vi "cm2nm_add_new_sample_point_to_session_array.vi"(4 "Sample Set":T2, 6 "Enter New Point":T1) -> (0 "XY_graphOut":cluster{dbl[], dbl[]}[](array[cluster]), 1 "NewPoint":T1={"MetaDataFile"=path "", "X"=nan, "Y"=nan, "Z"=0.0, "Group"=0, "Rotation"=0.0, "Fiducial"=FALSE, "Magnification"=0.0, "Working_Distance"=0.0, "Notes"="", "Location Name/ID"="", "OtherRelatedDataFiles"=[], "Available"=FALSE}, 2 "SetIndexOfarrytoEnd":i32[](array[numeric]), 3 "Sample Set Out":T2, 5 "Fiducial Count":u32[](array[colorbox]), 7 "List of Points":string[](array[string]))   [LabVIEW 2011]
uses:
  cm2nm_coordinate_information_v2.ctl
  cm2nm_sample_set.ctl
  Instrument_type_enum_v2.ctl
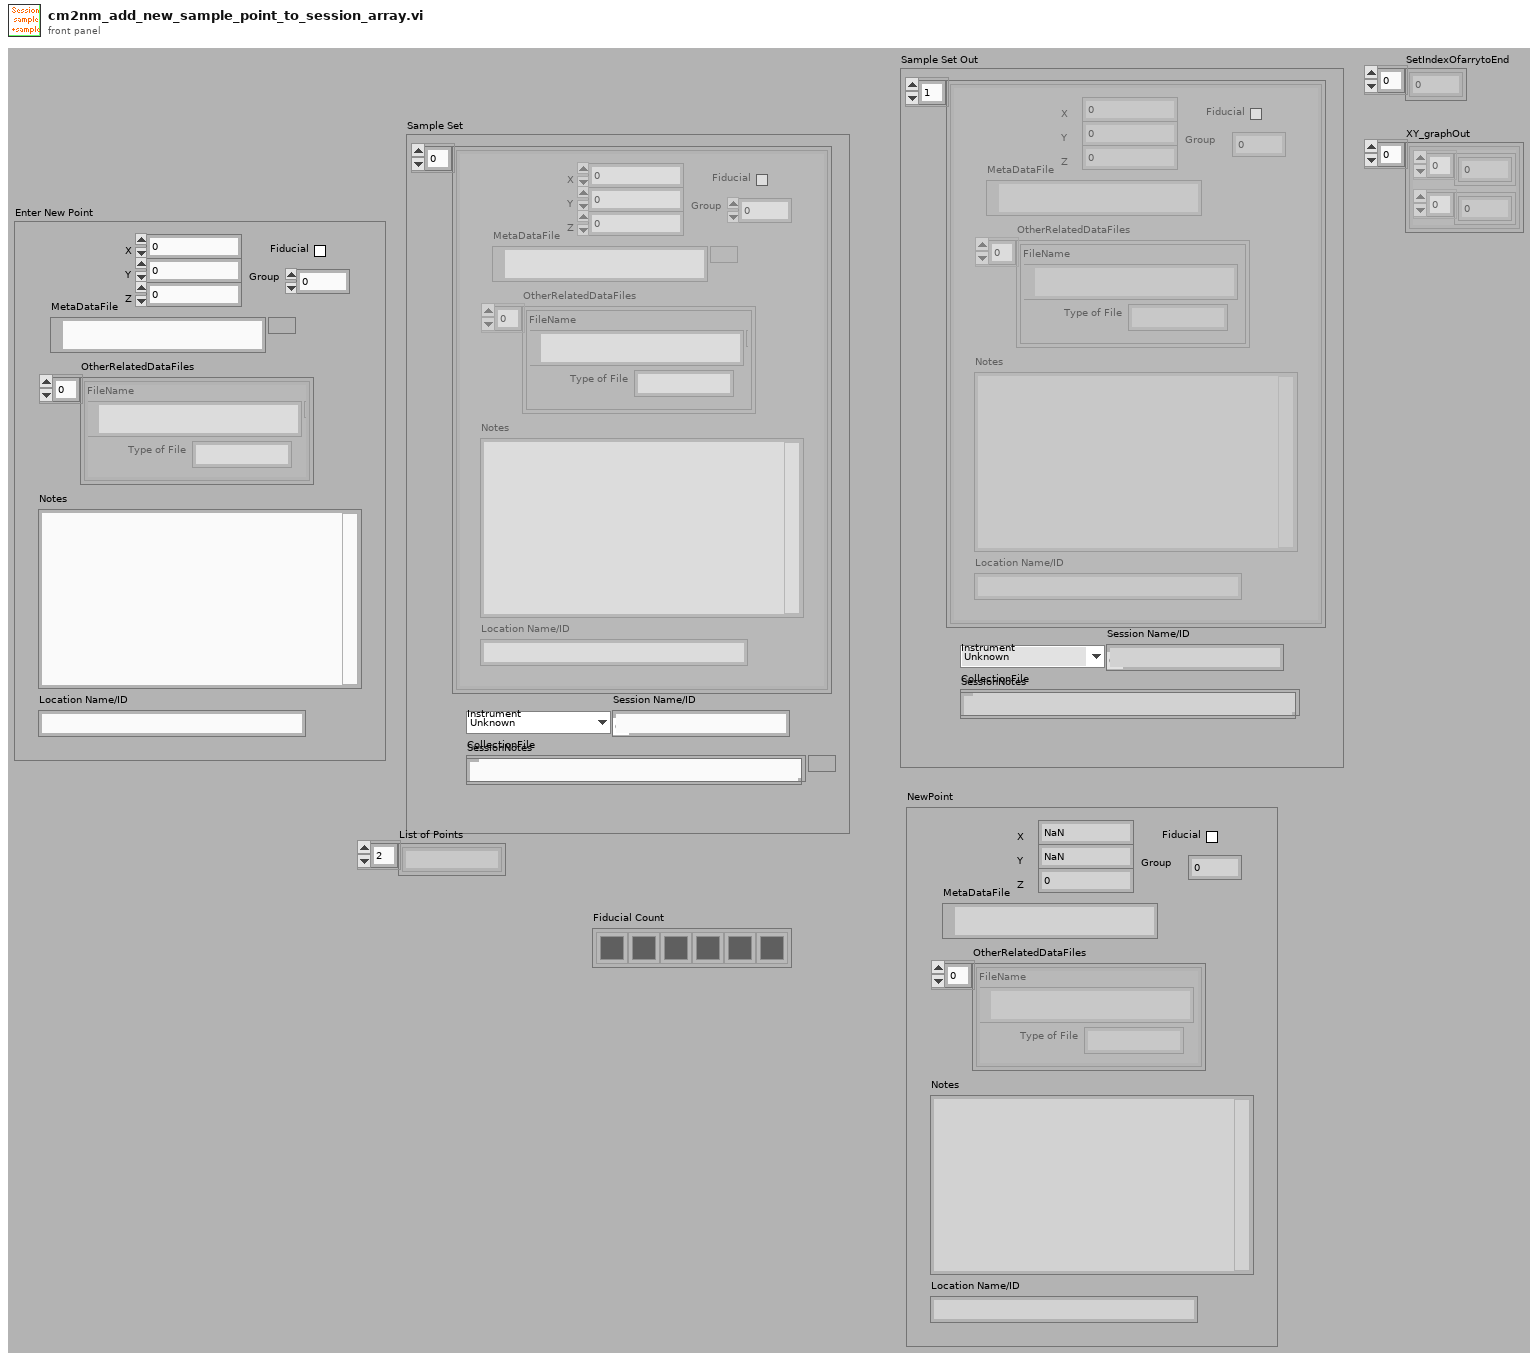
[diagram p1: front panel]
types:
  T1 = typedef "cm2nm_coordinate_information_v2.ctl" = cluster{"MetaDataFile":path, "X":dbl, "Y":dbl, "Z":dbl, "Group":i32, "Rotation":dbl[unit], "Fiducial":bool, "Magnification":dbl, "Working_Distance":dbl, "Notes":string, "Location Name/ID":string, "OtherRelatedDataFiles":cluster{"Type of File":string, "FileName":path}[], "Available":bool}
  T2 = typedef "cm2nm_sample_set.ctl" = cluster{"CollectionOfPoints":T1[], "Instrument":T3, "CollectionFile":path, "Session Name/ID":string, "SessionNotes":string}
  T3 = typedef "Instrument_type_enum_v2.ctl" = enum16{"Unknown", "Philips FEI SEM IRC", "JEOL 7000F EML_MFC", "MXRD MFC", "JEOL_EPMA"}
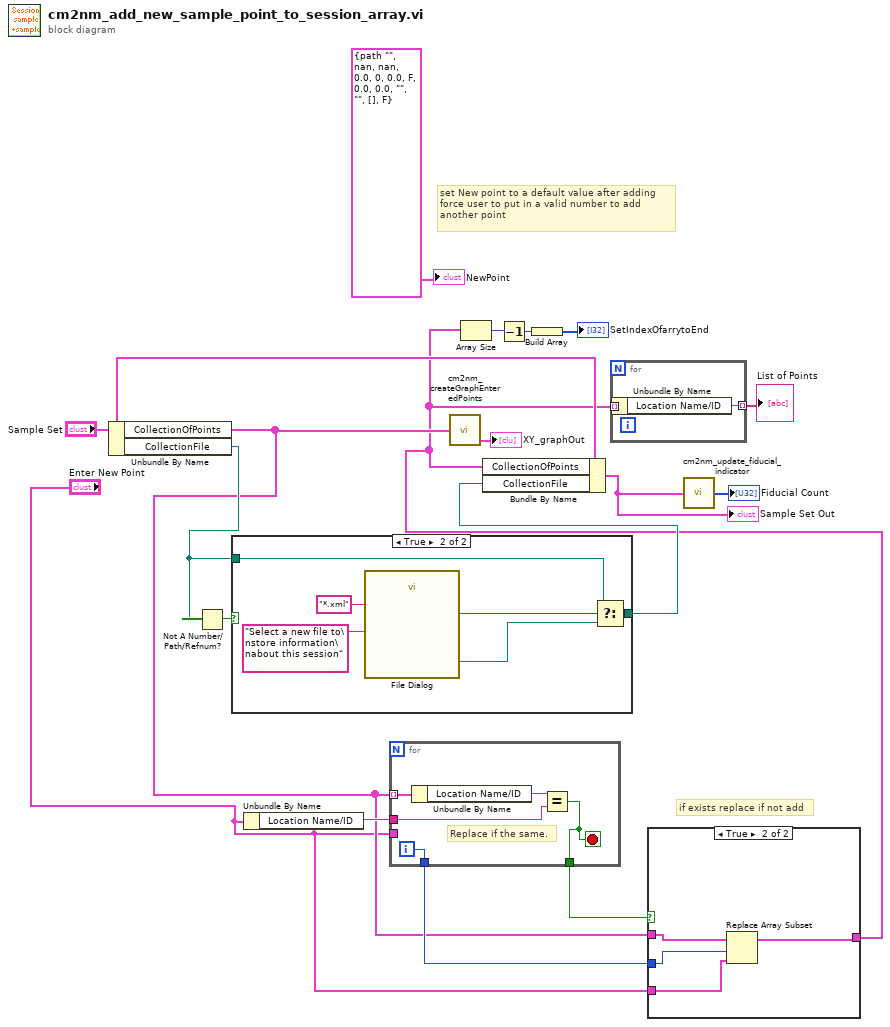
[diagram p0: block diagram]
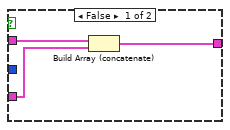
[diagram p2: hidden frame]
diagram:
  # "if exists replace if not add"
  # "set New point to a default value after adding\nforce user to put in a valid number to add\nanother point"
  n1 = Unbundle By Name("Sample Set") -> ("CollectionOfPoints"=w3:T1[], "CollectionFile"=w9:path)
  n2 = Not A Number/Path/Refnum?(number/path/refnum=w9) -> (NaN/Path/Refnum?=w10:bool)
  n3 = case shown="True" w10 {
    tunnel: w9 -> [w19 w20]
    tunnel: [w19 w21] -> w8
    frame False {
    }
    frame True {
      n4 = call "File Dialog"("prompt"="Select a new file to\nstore information\nabout this session", "pattern (all files)"="*.xml") -> ("selected path"=w22:path, "cancelled"=w23:bool)  [unwired: 5 in, 7 out]
      n5 = Select(t=w20, s=w23, f=w22) -> (s? t:f=w21:path)
    }
  }
  n6 = Unbundle By Name("Enter New Point") -> ("Location Name/ID"=w6:string)
  n7 = for {
    tunnel: w3 -> [w28] mode=indexing
    tunnel: w6 -> [w30]
    tunnel: "Enter New Point" -> [_]
    tunnel: [w27] -> w4
    tunnel: [w26] -> w5
    i -> [w27]
    stop <- w26 stop-if-true
    # "Replace if the same."
    n8 = Unbundle By Name(w28) -> ("Location Name/ID"=w29:string)
    n9 = Equal?(x=w29, y=w30) -> (x = y?=w26:bool)
  }
  n10 = call "cm2nm_createGraphEnteredPoints.vi"("EnteredPoints_in"=w3) -> ("XY_graphOut"=→"XY_graphOut":cluster{dbl[], dbl[]}[])
  n11 = case shown="True" w5 {
    tunnel: w4 -> [_ w36]
    tunnel: w3 -> [w33 w37]
    tunnel: "Enter New Point" -> [w32 w35]
    tunnel: [w31 w34] -> w1
    frame False {
      n12 = Build Array (concatenate)(w33, w32) -> (w31:T1[])
    }
    frame True {
      n13 = Replace Array Subset(array=w37, new element=w35, index=w36) -> (w34:T1[])
    }
  }
  n14 = Array Size(array=w1) -> (size(s)=w15:i32)
  n15 = Bundle By Name(cluster="Sample Set", "CollectionOfPoints"=w1, "CollectionFile"=w8) -> (w11:T2)
  "Sample Set Out" <- w11
  n16 = Decrement(x=w15) -> (x-1=w14:i32)
  n17 = Build Array(w14) -> (→"SetIndexOfarrytoEnd":i32[])
  n18 = for {
    tunnel: w1 -> [w39] mode=indexing
    tunnel: [w38] -> w7 mode=indexing
    n19 = Unbundle By Name(w39) -> ("Location Name/ID"=w38:string)
  }
  "List of Points" <- w7
  n20 = call "cm2nm_update_fiducial_indicator.vi"("Sample Set"=w11) -> ("Array"=→"Fiducial Count":u32[])
  "NewPoint" <- T1 {"MetaDataFile"=path "", "X"=nan, "Y"=nan, "Z"=0.0, "Group"=0, "Rotation"=0.0, "Fiducial"=FALSE, "Magnification"=0.0, "Working_Distance"=0.0, "Notes"="", "Location Name/ID"="", "OtherRelatedDataFiles"=[], "Available"=FALSE} ("Enter New Point")
